vi "Revision Query.vi"(0 "VISA resource name":refnum<visa-resource-name>, 11 "error in (no error)":errorcluster) -> (4 "VISA resource name out":refnum<visa-resource-name>, 6 "Instr Serial Number":string, 8 "Instr Driver Revision":string, 10 "Instr Firmware Revision":string, 14 "Instr Model Number":string, 15 "error out":errorcluster)   [LabVIEW 2019, in "Lake Shore Cryotronics 370.lvlib"]
doc: "This VI queries the current instrument firmware revision and instrument driver revision.\nThis Instrument Driver's Revision number is \"REV 1.0, 05/2001, LV 5.0\" and is compatible with Instrument Firmware Revision: \"M370F 03/30/01\" and later.\n\nLakeShore Cryotronics Model 370 AC Resistance Bridge\nCreated By: Rob Welsh\nRelease Date: May 2001\nOriginally Developed in LabVIEW Version: 5.0\n\nModification History: \n\nNone"
uses:
  Lake Shore Cryotronics 370.lvlib
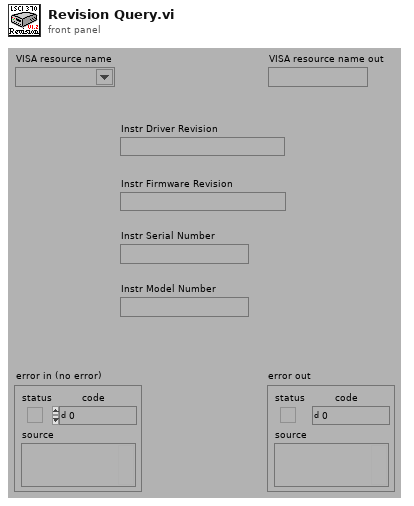
[diagram p1: front panel]
types:
  T1 = enum32{"invalid app kind", "Development System", "Run Time System", "Student Edition", "Embedded LabVIEW", "Evaluation", "Custom"}
  T2 = cluster{"Major":u16, "Minor":u16, "Fix":u16, "Build":u16}
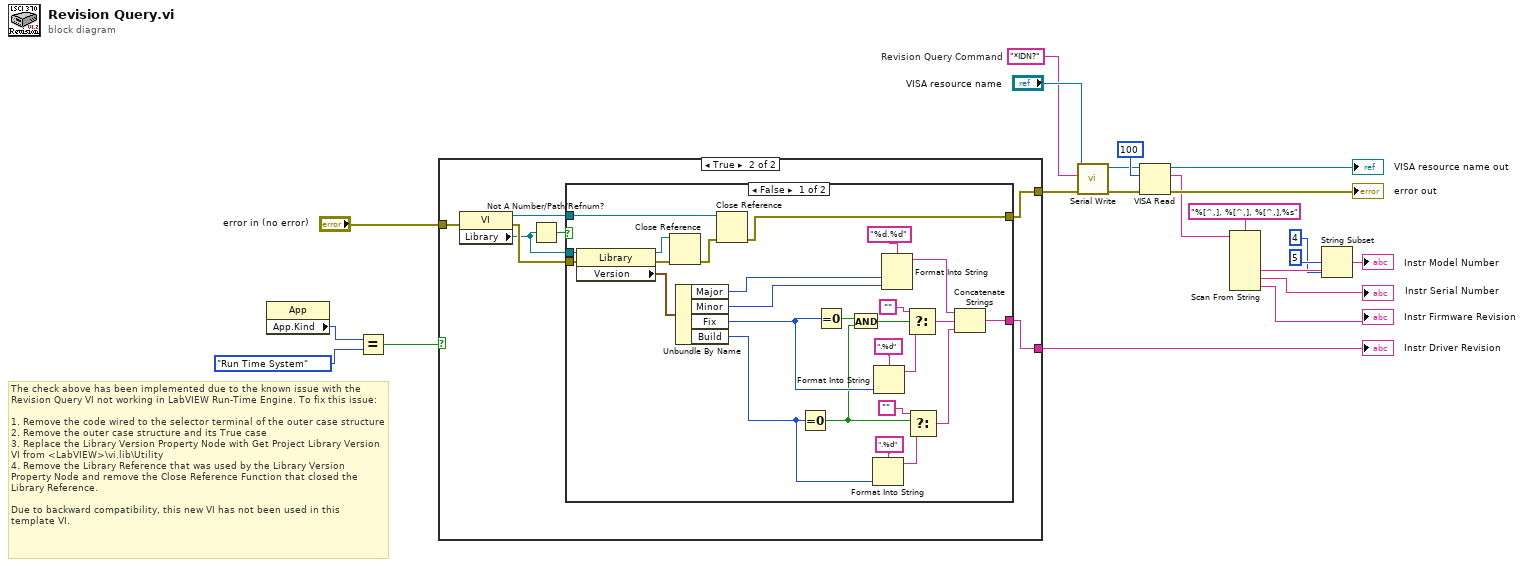
[diagram p0: block diagram]
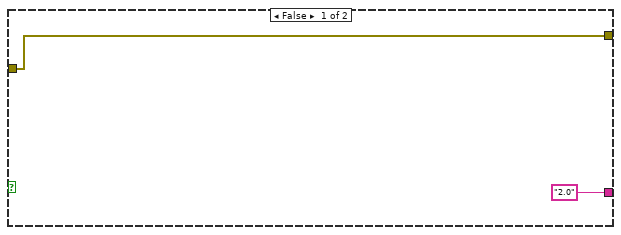
[diagram p2: hidden frame]
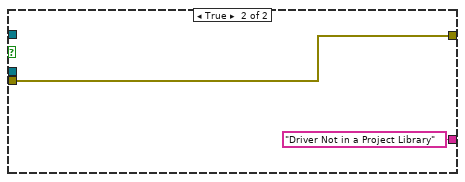
[diagram p3: hidden frame]
diagram:
  w15 = "*IDN?"  # Revision Query Command
  # "The check above has been implemented due to the known issue with the Revision Query VI not working in LabVIEW Run-Time Engine. To fix this issue:\n\n1. Remove the code wired to the selector terminal of the outer case structure\n2. Remove the outer case structure and its True case\n3. Replace the Library Version Property Node with Get Project Library Version VI from <LabVIEW>\\vi.lib\\Utility\n4. Remove the Library Reference that was used by the Library Version Property Node and remove the Close Reference Function that closed the Library Reference.\n\nDue to backward compatibility, this new VI has not been used in this template VI."
  n1 = property class="App"() -> ("App.Kind"=w3:T1)  [unwired: 2 in, 2 out]
  n2 = Equal?(x=w3, y=T1."Run Time System" ("Application:Kind")) -> (x = y?=w1:bool)
  n3 = case shown="True" w1 {
    tunnel: ["2.0" w26] -> w6
    tunnel: "error in (no error)" -> [w23 w25]
    tunnel: [w23 w24] -> w4
    frame False {
    }
    frame True {
      n4 = property class="VI"(error in=w25) -> (reference out=w30:refnum<vi>, error out=w29:errorcluster, "Library"=w28:refnum<vi>)  [unwired: 1 in]
      n5 = Not A Number/Path/Refnum?(number/path/refnum=w28) -> (NaN/Path/Refnum?=w27:bool)
      n6 = case shown="False" w27 {
        tunnel: w30 -> [w53 _]
        tunnel: w29 -> [w40 w58]
        tunnel: [w36 w58] -> w24
        tunnel: [w35 "Driver Not in a Project Library"] -> w26
        tunnel: w28 -> [w34 _]
        frame False {
          n7 = property class="Library"(reference=w34, error in=w40) -> (reference out=w55:refnum<vi>, error out=w56:errorcluster, "Version"=w52:T2)
          n8 = Close Reference(reference=w55, error in (no error)=w56) -> (error out=w54:errorcluster)
          n9 = Unbundle By Name(w52) -> ("Major"=w43:u16, "Minor"=w42:u16, "Fix"=w39:u16, "Build"=w41:u16)
          n10 = Close Reference(reference=w53, error in (no error)=w54) -> (error out=w36:errorcluster)
          n11 = Equal To 0?(x=w41) -> (x = 0?=w32:bool)
          n12 = Equal To 0?(x=w39) -> (x = 0?=w38:bool)
          n13 = And(x=w38, y=w32) -> (x .and. y?=w37:bool)
          n14 = Format Into String(format string=".%d", w41) -> (resulting string=w46:string)  [unwired: 2 in, 1 out]
          n15 = Format Into String(format string=".%d", w39) -> (resulting string=w50:string)  [unwired: 2 in, 1 out]
          n16 = Format Into String(format string="%d.%d", w43, w42) -> (resulting string=w48:string)  [unwired: 2 in, 1 out]
          n17 = Select(t="", s=w37, f=w50) -> (s? t:f=w47:string)
          n18 = Select(t="", s=w32, f=w46) -> (s? t:f=w44:string)
          n19 = Concatenate Strings(w48, w47, w44) -> (w35:string)
        }
        frame True {
        }
      }
    }
  }
  "Instr Driver Revision" <- w6
  n20 = call "Serial Write.vi"("error in (no error)"=w4, "Write Buffer (\"\")"=w15, "VISA resource name"="VISA resource name") -> ("error out"=w16:errorcluster, "VISA resource name out"=w17:refnum<visa-resource-name>)  [unwired: 6 in, 1 out]
  n21 = VISA Read(VISA resource name=w17, byte count=u32 100 ("Num Bytes to Read"), error in (no error)=w16) -> (VISA resource name out=→"VISA resource name out":refnum<visa-resource-name>, read buffer=w10:string, error out=→"error out":errorcluster)  [unwired: 1 out]
  n22 = Scan From String(format string="%[^,], %[^,], %[^,],%s", input string=w10) -> (output 2=w13:string, output 3=→"Instr Serial Number":string, output 4=→"Instr Firmware Revision":string)  [unwired: 7 in, 3 out]
  n23 = String Subset(string=w13, offset (0)=5, length (rest)=4) -> (substring=→"Instr Model Number":string)
